vi "Custom Gyro Drive.vi"(0 "RobotDriveDevRef":T8={"DevStatus"={"status"=FALSE, "code"=0, "source"=""}, "Motors[]"=[], "Square Inputs"=FALSE, "Max Output"=1.0}, 5 "Left Joystick":dbl, 7 "Gyro Correction":bool, 9 "Right Joystick":dbl, 11 "error in (no error)":errorcluster) -> (4 "RobotDriveDevRef 2":T8={"DevStatus"={"status"=FALSE, "code"=0, "source"=""}, "Motors[]"=[], "Square Inputs"=FALSE, "Max Output"=1.0}, 6 "Middle Left Motor":T1={"DeviceStatus"={"status"=FALSE, "code"=0, "source"=""}, "Type"=enum."PWM", "PWM"={"PWM Channel"=enum."PWM 1", "DeadBand"={"Name"="", "maxPositivePwm"=0, "minPositivePwm"=0, "centerPwm"=0, "maxNegativePwm"=0, "minNegativePwm"=0, "angularRange"=0}}, "CAN"={"Device Number"=0, "Control Mode"=enum."Percent VBus", "Semaphore"=refnum, "Max Vout"=12.0, "TalonSRX Control Mode"=enum."Percent VBus"}, "Invert"=FALSE}, 8 "Middle Right Motor":T1={"DeviceStatus"={"status"=FALSE, "code"=0, "source"=""}, "Type"=enum."PWM", "PWM"={"PWM Channel"=enum."PWM 1", "DeadBand"={"Name"="", "maxPositivePwm"=0, "minPositivePwm"=0, "centerPwm"=0, "maxNegativePwm"=0, "minNegativePwm"=0, "angularRange"=0}}, "CAN"={"Device Number"=0, "Control Mode"=enum."Percent VBus", "Semaphore"=refnum, "Max Vout"=12.0, "TalonSRX Control Mode"=enum."Percent VBus"}, "Invert"=FALSE}, 10 "Motor Values":dbl[](array[numeric]), 15 "error out":errorcluster)   [LabVIEW 2015]
uses:
  <vilib>/Rock Robotics/WPI/RobotDrive/WPI_RobotDriveDevRef.ctl
  <vilib>/Rock Robotics/WPI/MotorControl/WPI_MotorControlDeviceRef.ctl
  <vilib>/Rock Robotics/WPI/MotorControl/WPI_MotorControlType.ctl
  <vilib>/Rock Robotics/SystemInterfaces/DIO/FPGA_DIOPWMChannel.ctl
  <vilib>/Rock Robotics/WPI/PWM/WPI_PWMDeadband.ctl
  <vilib>/Rock Robotics/WPI/CAN/Jaguar/SubVIs/WPI_CANJaguar_ControlMode.ctl
  <vilib>/Rock Robotics/WPI/CAN/TalonSRX/WPI_CANTalonSRX_APIControlMode.ctl
  <vilib>/Rock Robotics/SystemInterfaces/NetworkCommunication/NetComm_UsageReport_ResourceType.ctl
  Robot Global Data.vi
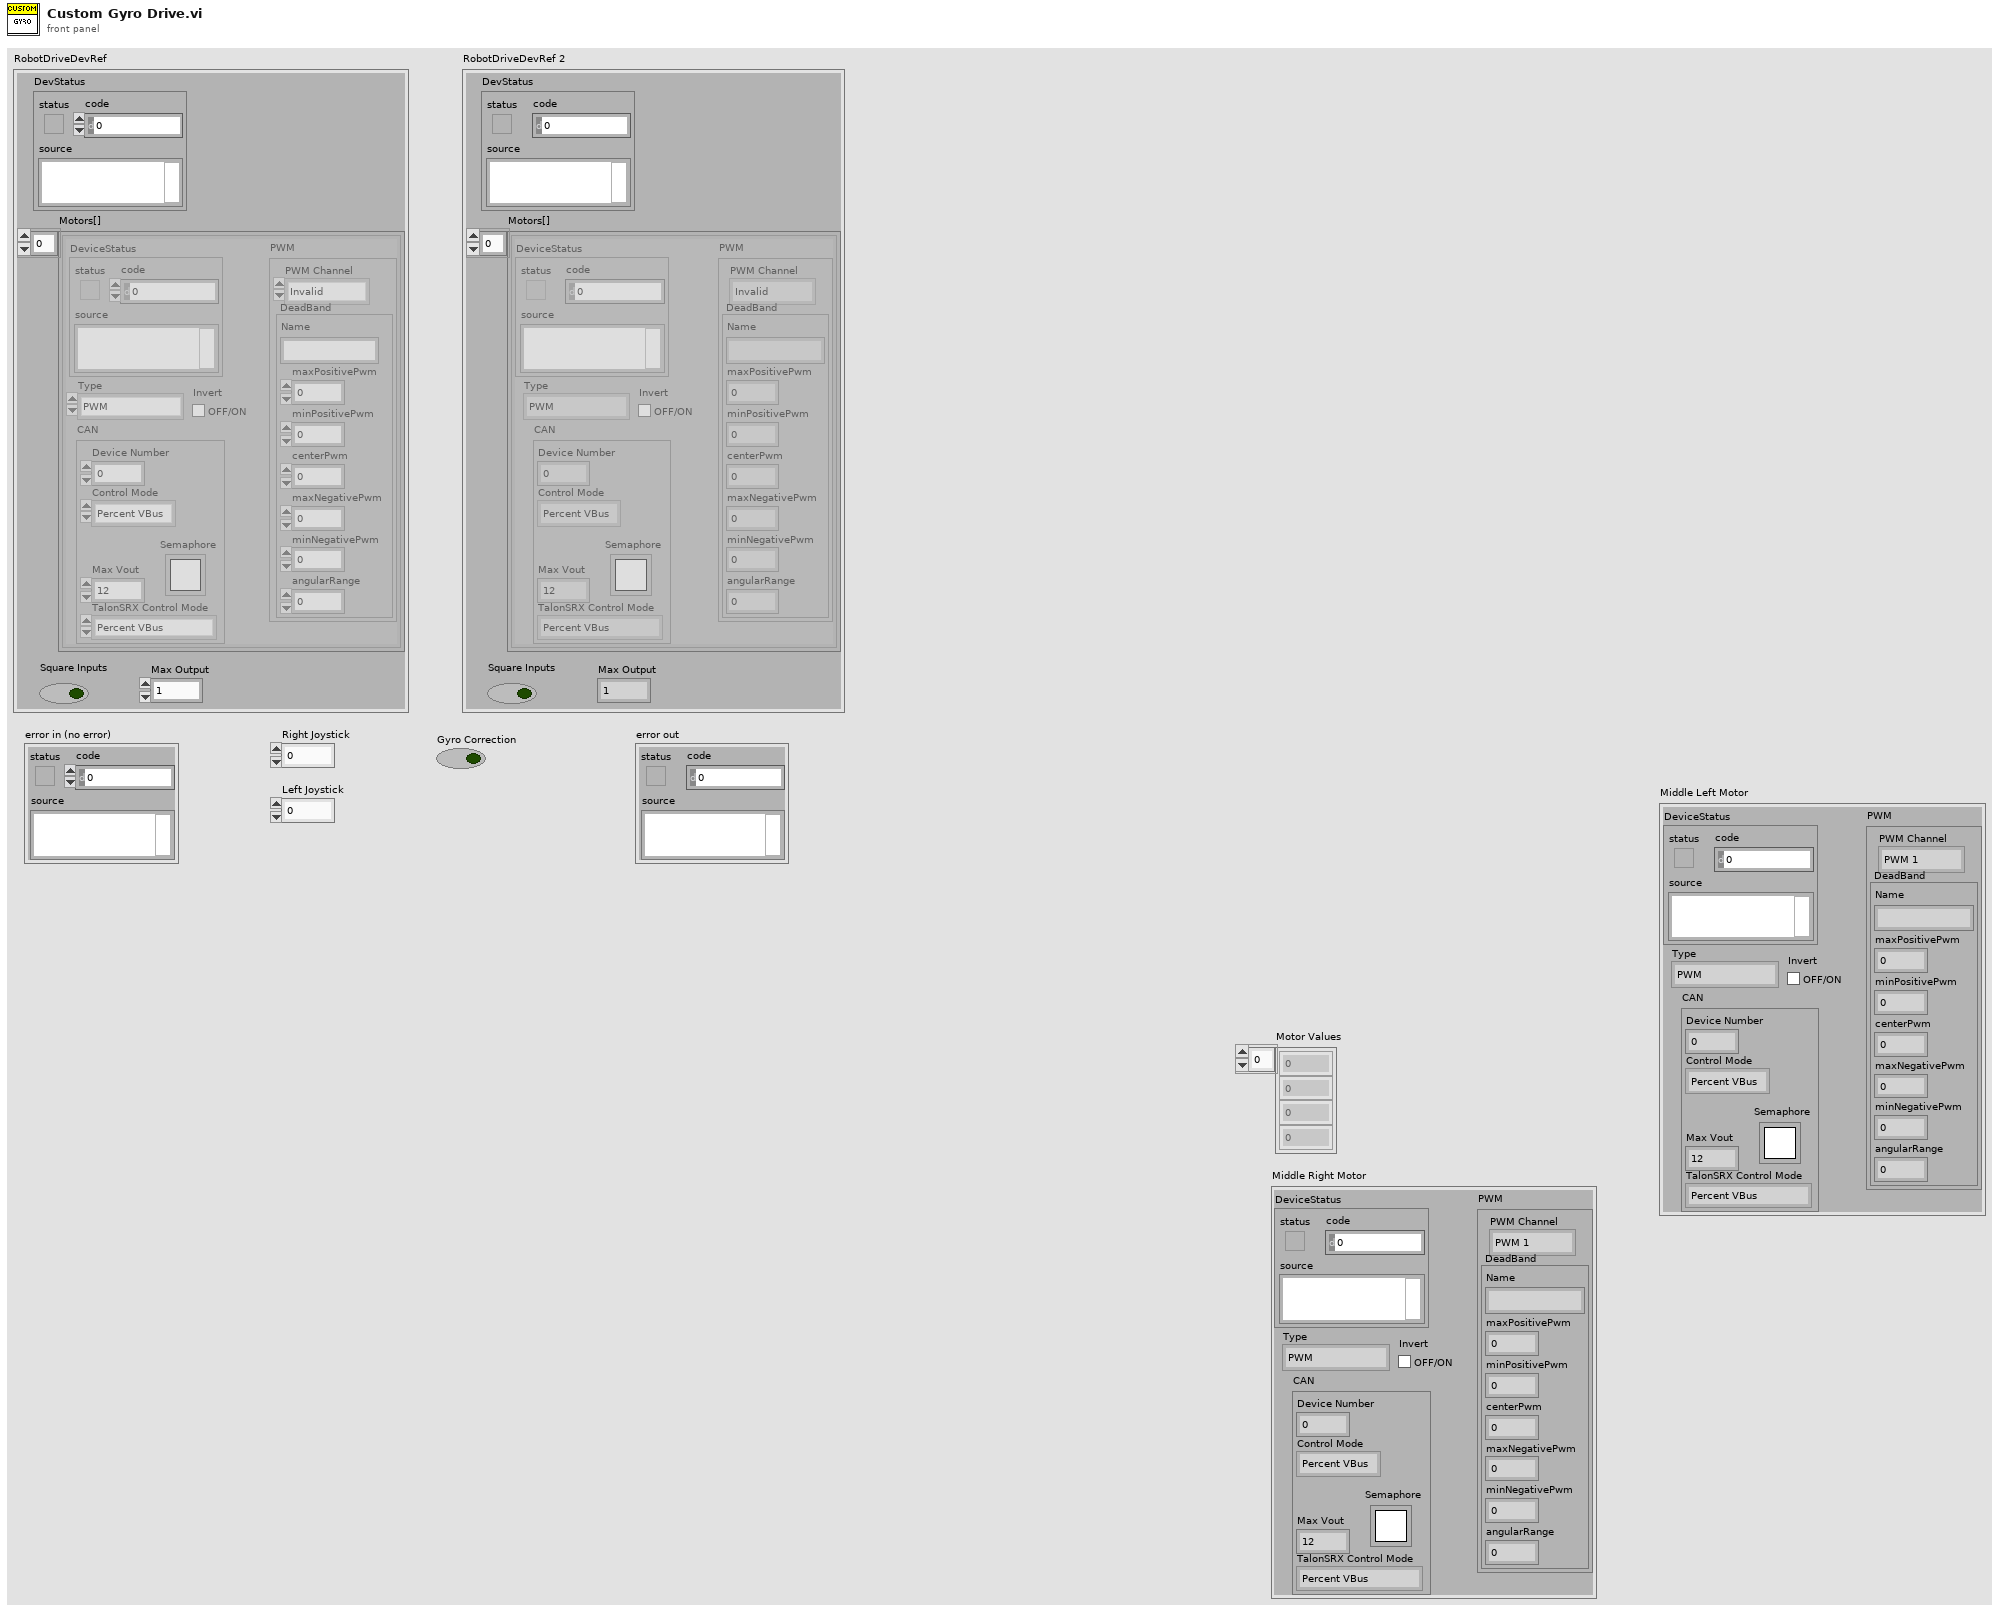
[diagram p1: front panel]
types:
  T1 = typedef "WPI_MotorControlDeviceRef.ctl" = cluster{"DeviceStatus":errorcluster, "Type":T2, "PWM":cluster{"PWM Channel":T3, "DeadBand":T4}, "CAN":cluster{"Device Number":u8, "Control Mode":T5, "Semaphore":T6, "Max Vout":dbl, "TalonSRX Control Mode":T7}, "Invert":bool}
  T2 = typedef "WPI_MotorControlType.ctl" = enum16{"PWM", "CAN", "CANTalonSRX"}
  T3 = typedef "FPGA_DIOPWMChannel.ctl" = enum8{"PWM 0", "PWM 1", "PWM 2", "PWM 3", "PWM 4", "PWM 5", "PWM 6", "PWM 7", "PWM 8", "PWM 9", "PWM MXP 0", "PWM MXP 1", "PWM MXP 2", "PWM MXP 3", "PWM MXP 4", "PWM MXP 5", "PWM MXP 6", "PWM MXP 7", "PWM MXP 8", "PWM MXP 9", "Invalid"}
  T4 = typedef "WPI_PWMDeadband.ctl" = cluster{"Name":string, "maxPositivePwm":i32, "minPositivePwm":i32, "centerPwm":i32, "maxNegativePwm":i32, "minNegativePwm":i32, "angularRange":u16}
  T5 = typedef "WPI_CANJaguar_ControlMode.ctl" = enum8{"Percent VBus", "Current", "Speed", "Position", "Voltage"}
  T6 = typedef "Semaphore RefNum" = refnum<k1>
  T7 = typedef "WPI_CANTalonSRX_APIControlMode.ctl" = enum8{"Percent VBus", "Speed", "Position", "Slave", "Unchanged / Invalid", "Voltage Compensation", "Current", "Motion Profile"}
  T8 = typedef "WPI_RobotDriveDevRef.ctl" = cluster{"DevStatus":errorcluster, "Motors[]":T1[], "Square Inputs":bool, "Max Output":dbl}
  T9 = typedef "NetComm_UsageReport_ResourceType.ctl" = enum8{"Controller", "Module", "Language", "CANPlugin", "Accelerometer", "ADXL345", "AnalogChannel", "AnalogTrigger", "AnalogTriggerOutput", "CANJaguar", "Compressor", "Counter", "Dashboard", "DigitalInput", "DigitalOutput", "DriverStationCIO", "DriverStationEIO", "DriverStationLCD", "Encoder", "GearTooth", "Gyro", "I2C", "Framework", "Jaguar", "Joystick", "Kinect", "KinectStick", "PIDController", "Preferences", "PWM", "Relay", "RobotDrive", "SerialPort", "Servo", "Solenoid", "SPI", "Task", "Ultrasonic", "Victor", "Button", "Command", "AxisCamera", "PCVideoServer", "SmartDashboard", "Talon", "HiTechnicColorSensor", "HiTechnicAccel", "HiTechnicCompass", "SRF08", "AnalogOutput", "Victor SP", "Talon SRX", "CAN Talon SRX", "ADXL362 Accel", "ADXRS450 Gyro", "Rev SPARK", "Mindsensors SD540", "Digital Filter"}
  T10 = typedef "WPI_GyroDevRef.ctl" = cluster{"DevStatus":errorcluster, "Analog Channel":T11, "Offset":dbl, "Gain (VoltsPerDegree/Second)":dbl, "Gyro Type":enum16{"Analog", "XRS450"}, "Handle":i32, "SPI Bus":T12, "Device Found":bool, "Sample Rate":dbl, "Calibrate On Open":bool}
  T11 = typedef "FPGA_AIChannel.ctl" = enum8{"AI 0", "AI 1", "AI 2", "AI 3", "AI MXP 0", "AI MXP 1", "AI MXP 2", "AI MXP 3", "Invalid"}
  T12 = typedef "spi_bus.ctl" = enum16{"SPI On-Board, CS0", "SPI On-Board, CS1", "SPI On-Board, CS2", "SPI On-Board, CS3", "SPI MXP", "Invalid"}
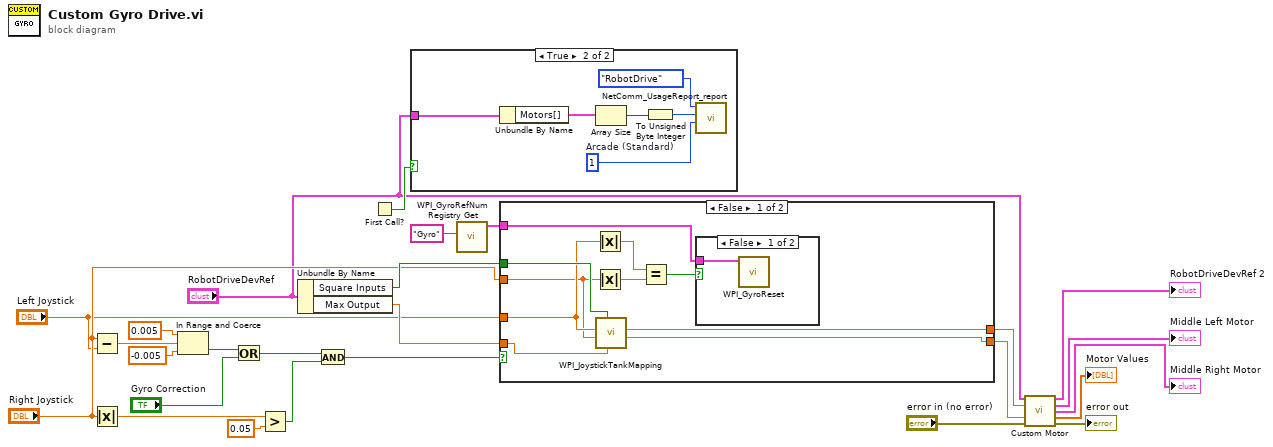
[diagram p0: block diagram]
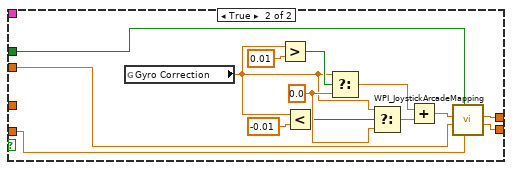
[diagram p3: hidden frame]
diagram:
  n1 = Subtract(x="Right Joystick", y="Left Joystick") -> (x-y=w11:dbl)
  n2 = Absolute Value(x="Right Joystick") -> (abs(x)=w16:dbl)
  n3 = In Range and Coerce(upper limit=0.005, x=w11, lower limit=-0.005) -> (In Range?=w21:bool)  [unwired: 1 out]
  n4 = Or(x=w21, y="Gyro Correction") -> (x .or. y?=w19:bool)
  n5 = Greater?(x=w16, y=0.05 ("x")) -> (0:w17:bool)
  n6 = Unbundle By Name("RobotDriveDevRef") -> ("Square Inputs"=w24:bool, "Max Output"=w25:dbl)
  n7 = And(x=w19, y=w17) -> (x .and. y?=w18:bool)
  n8 = First Call?() -> (First Call?: T/F=w26:bool)
  n9 = case shown="True" w26 {
    tunnel: "RobotDriveDevRef" -> [_ w28]
    frame False {
    }
    frame True {
      w30 = u8 1  # Arcade (Standard)
      n10 = Unbundle By Name(w28) -> ("Motors[]"=w27:T1[])
      n11 = Array Size(array=w27) -> (size(s)=w29:i32)
      n12 = To Unsigned Byte Integer(number=w29) -> (unsigned 8bit integer=w31:u8)
      n13 = call <vilib>:"NetComm_UsageReport_report.vi"("Context"=w30, "Instance Number"=w31, "Resource Type"=NetComm_UsageReport_ResourceType."RobotDrive") -> ()  [unwired: 9 in]
    }
  }
  n14 = call <vilib>:"WPI_GyroRefNum Registry Get.vi"("refnum name"="Gyro") -> ("GyroDevRef"=w14:T10)  [unwired: 9 in, 1 out]
  n15 = case shown="False" w18 {
    tunnel: [w42 w48] -> w9
    tunnel: [w41 w57] -> w8
    tunnel: "Right Joystick" -> [w36 w45]
    tunnel: w25 -> [w40 w47]
    tunnel: w24 -> [w39 w46]
    tunnel: w14 -> [w38 _]
    tunnel: "Left Joystick" -> [w37 _]
    frame False {
      n16 = Absolute Value(x=w37) -> (abs(x)=w35:dbl)
      n17 = Absolute Value(x=w36) -> (abs(x)=w34:dbl)
      n18 = call <vilib>:"WPI_JoystickTankMapping.vi"("Max Output"=w40, "Square Inputs"=w39, "Right axis value"=w36, "Left axis value"=w37) -> ("Right Motor Value"=w41:dbl, "Left Motor Value"=w42:dbl)  [unwired: 6 in]
      n19 = Equal?(x=w35, y=w34) -> (x = y?=w33:bool)
      n20 = case shown="False" w33 {
        tunnel: w38 -> [w43 _]
        frame False {
          n21 = call <vilib>:"WPI_GyroReset.vi"("GyroDevRef"=w43) -> ()  [unwired: 9 in, 2 out]
        }
        frame True {
        }
      }
    }
    frame True {
      w56 = 0.0 ("f")
      n22 = global read "Robot Global Data.vi" "Gyro Correction"() -> (w44:dbl)
      n23 = Greater?(x=w44, y=0.01) -> (0:w54:bool)
      n24 = Less?(x=w44, y=-0.01) -> (x < y?=w55:bool)
      n25 = Select(t=w44, s=w54, f=w56) -> (s? t:f=w51:dbl)
      n26 = Select(t=w44, s=w55, f=w56) -> (s? t:f=w50:dbl)
      n27 = Add(x=w51, y=w50) -> (x+y=w49:dbl)
      n28 = call <vilib>:"WPI_JoystickArcadeMapping.vi"("Max Output"=w47, "Square Inputs"=w46, "Y axis value"=w45, "X axis value"=w49) -> ("Right Motor Value"=w57:dbl, "Left Motor Value"=w48:dbl)  [unwired: 6 in]
    }
  }
  n29 = call "Custom Motor.vi"("RobotDriveDevRef in"="RobotDriveDevRef", "LeftSpeed"=w9, "RightSpeed"=w8, "error in (no error)"="error in (no error)") -> ("RobotDriveDevRef out"=→"RobotDriveDevRef 2":T8, "Middle Left Motor"=→"Middle Left Motor":T1, "Middle Right Motor"=→"Middle Right Motor":T1, "Motor Values"=→"Motor Values":dbl[], "error out"=→"error out":errorcluster)  [unwired: 7 in]
